vi "writeHeader.vi"(8 "error in (no error)":errorcluster, 9 "Length":u16, 10 "Subnet":u8, 11 "ModbusBuffer in":refnum<class "ModbusBuffer.lvclass">) -> (0 "error out":errorcluster, 3 "ModbusBuffer out":refnum<class "ModbusBuffer.lvclass">)   [LabVIEW 2016, in "RTModbus.lvlib" / "ModbusBuffer.lvclass"]
uses:
  ModbusBuffer.lvclass
  ModbusBuffer.lvclass/ModbusBuffer.ctl
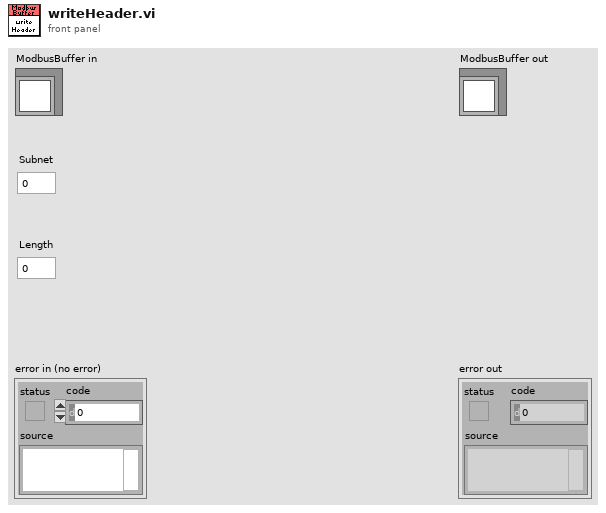
[diagram p1: front panel]
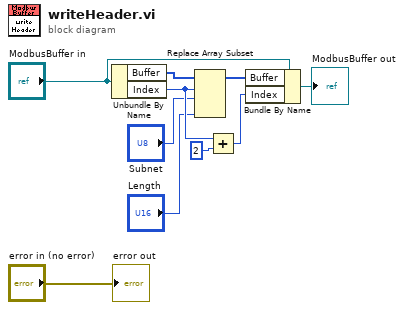
[diagram p0: block diagram]
diagram:
  n1 = Unbundle By Name("ModbusBuffer in") -> ("Buffer"=w6:u16[], "Index"=w5:i32)
  n2 = Replace Array Subset(array=w6, new element #1="Subnet", index #1=w5, new element #2="Length") -> (w8:u16[])  [unwired: 1 in]
  n3 = Add(x=w5, y=2) -> (x+y=w9:i32)
  n4 = Bundle By Name(cluster="ModbusBuffer in", "Buffer"=w8, "Index"=w9) -> (→"ModbusBuffer out":refnum<class "ModbusBuffer.lvclass">)
  "error out" <- "error in (no error)"
